vi "user32_DrawIcon.vi"(0 "hDC":u32, 5 "Position":cluster{"x":i32, "y":i32}, 7 "hIcon":u32, 11 "错误输入（无错误）":errorcluster) -> (4 "dup hDC":u32, 6 "success?":bool, 15 "错误输出":errorcluster)   [LabVIEW 2011]
doc: "该函数在限定的设备上下文窗口的客户区域绘制图标。"
uses:
  user32.dll
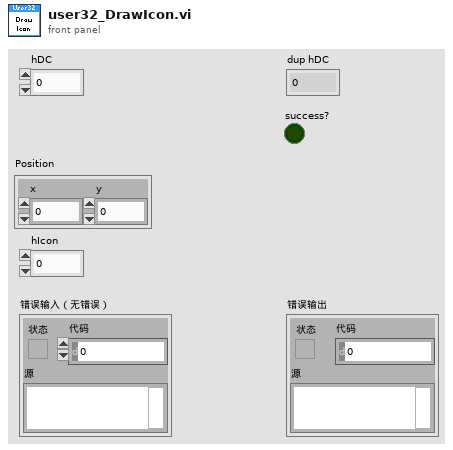
[diagram p1: front panel]
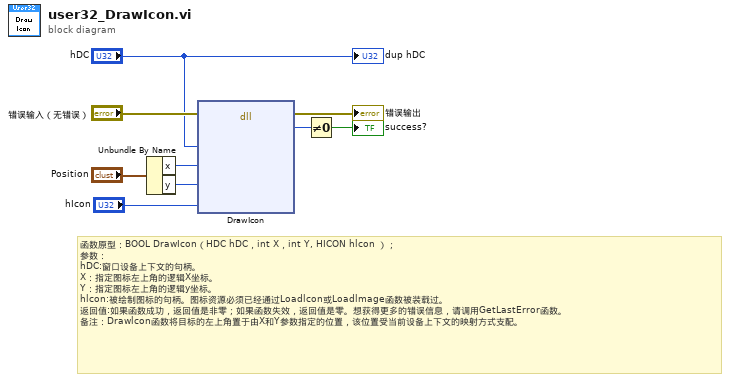
[diagram p0: block diagram]
diagram:
  # "函数原型：BOOL DrawIcon（HDC hDC，int X，int Y, HICON hlcon ）；\n参数：\nhDC:窗口设备上下文的句柄。\nX：指定图标左上角的逻辑X坐标。\nY：指定图标左上角的逻辑y坐标。\nhlcon:被绘制图标的句柄。图标资源必须已经通过Loadlcon或Loadlmage函数被装载过。\n返回值:如果函数成功，返回值是非零；如果函数失效，返回值是零。想获得更多的错误信息，请调用GetLastError函数。\n备注：Drawlcon函数将目标的左上角置于由X和Y参数指定的位置，该位置受当前设备上下文的映射方式支配。"
  n1 = Unbundle By Name("Position") -> ("x"=w3:i32, "y"=w2:i32)
  n2 = dll-call lib="user32.dll" fn="DrawIcon"(error in="错误输入（无错误）", "hDC"="hDC", "x"=w3, "y"=w2, "hIcon"="hIcon") -> (error out=→"错误输出":errorcluster, "Bool"=w6:u8)  [unwired: 6 in, 1 out]
  n3 = Not Equal To 0?(x=w6) -> (x != 0?=→"success?":bool)
  "dup hDC" <- "hDC"
